vi "Corner Pixmap.vi"(10 "Corner":T2) -> (2 "Corner Pixmap":T1)   [LabVIEW 2022 SP3, in "FlexBlocks Support.lvlib"]
uses:
  FlexBlocks Support.lvlib
  <vilib>/picture/picture.llb/imagedata.ctl
  Corner.ctl
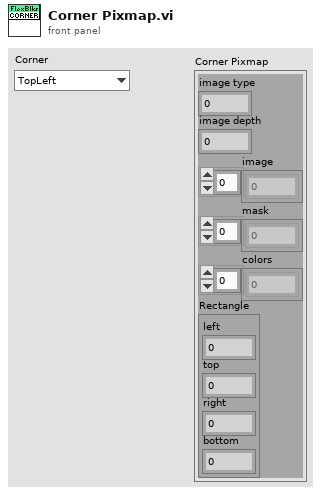
[diagram p1: front panel]
types:
  T1 = typedef "imagedata.ctl" = cluster{"image type":i32, "image depth":i32, "image":u8[], "mask":u8[], "colors":u32[], "Rectangle":cluster{"left":i16, "top":i16, "right":i16, "bottom":i16}}
  T2 = typedef "FlexBlocks Support.lvlib/Corner.ctl" = enum16{"TopLeft", "TopRight", "BottomLeft", "BottomRight"}
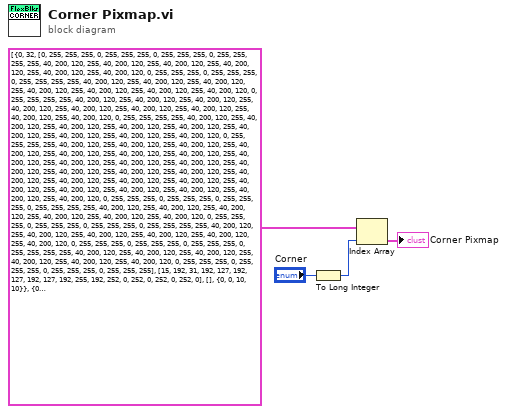
[diagram p0: block diagram]
diagram:
  n1 = To Long Integer(number="Corner") -> (32bit integer=w2:i32)
  n2 = Index Array(array=T1[] [{"image type"=0, "image depth"=32, "image"=[0, 255, 255, 255, 0, 255, 255, 255, 0, 255, 255, 255, 0, 255, 255, 255, 255, 40, 200, 120, 255, 40, 200, 120, 255, 40, 200, 120, 255, 40, 200, 120, 255, 40, 200, 120, 255, 40, 200, 120, 0, 255, 255, 255, 0, 255, 255, 255, 0, 255, 255, 255, 255, 40, 200, 120, 255, 40, 200, 120, 255, 40, 200, 120, 255, 40, 200, 120, 255, 40, 200, 120, 255, 40, 200, 120, 255, 40, 200, 120, 0, 255, 255, 255, 255, 40, 200, 120, 255, 40, 200, 120, 255, 40, 200, 120, 255, 40, 200, 120, 255, 40, 200, 120, 255, 40, 200, 120, 255, 40, 200, 120, 255, 40, 200, 120, 255, 40, 200, 120, 0, 255, 255, 255, 255, 40, 200, 120, 255, 40, 200, 120, 255, 40, 200, 120, 255, 40, 200, 120, 255, 40, 200, 120, 255, 40, 200, 120, 255, 40, 200, 120, 255, 40, 200, 120, 255, 40, 200, 120, 0, 255, 255, 255, 255, 40, 200, 120, 255, 40, 200, 120, 255, 40, 200, 120, 255, 40, 200, 120, 255, 40, 200, 120, 255, 40, 200, 120, 255, 40, 200, 120, 255, 40, 200, 120, 255, 40, 200, 120, 255, 40, 200, 120, 255, 40, 200, 120, 255, 40, 200, 120, 255, 40, 200, 120, 255, 40, 200, 120, 255, 40, 200, 120, 255, 40, 200, 120, 255, 40, 200, 120, 255, 40, 200, 120, 255, 40, 200, 120, 255, 40, 200, 120, 255, 40, 200, 120, 255, 40, 200, 120, 255, 40, 200, 120, 255, 40, 200, 120, 255, 40, 200, 120, 0, 255, 255, 255, 0, 255, 255, 255, 0, 255, 255, 255, 0, 255, 255, 255, 255, 40, 200, 120, 255, 40, 200, 120, 255, 40, 200, 120, 255, 40, 200, 120, 255, 40, 200, 120, 255, 40, 200, 120, 0, 255, 255, 255, 0, 255, 255, 255, 0, 255, 255, 255, 0, 255, 255, 255, 255, 40, 200, 120, 255, 40, 200, 120, 255, 40, 200, 120, 255, 40, 200, 120, 255, 40, 200, 120, 255, 40, 200, 120, 0, 255, 255, 255, 0, 255, 255, 255, 0, 255, 255, 255, 0, 255, 255, 255, 255, 40, 200, 120, 255, 40, 200, 120, 255, 40, 200, 120, 255, 40, 200, 120, 255, 40, 200, 120, 255, 40, 200, 120, 0, 255, 255, 255, 0, 255, 255, 255, 0, 255, 255, 255, 0, 255, 255, 255], "mask"=[15, 192, 31, 192, 127, 192, 127, 192, 127, 192, 255, 192, 252, 0, 252, 0, 252, 0, 252, 0], "colors"=[], "Rectangle"={"left"=0, "top"=0, "right"=10, "bottom"=10}}, {"image type"=0, "image depth"=32, "image"=[255, 40, 200, 120, 255, 40, 200, 120, 255, 40, 200, 120, 255, 40, 200, 120, 255, 40, 200, 120, 255, 40, 200, 120, 0, 255, 255, 255, 0, 255, 255, 255, 0, 255, 255, 255, 0, 255, 255, 255, 255, 40, 200, 120, 255, 40, 200, 120, 255, 40, 200, 120, 255, 40, 200, 120, 255, 40, 200, 120, 255, 40, 200, 120, 255, 40, 200, 120, 0, 255, 255, 255, 0, 255, 255, 255, 0, 255, 255, 255, 255, 40, 200, 120, 255, 40, 200, 120, 255, 40, 200, 120, 255, 40, 200, 120, 255, 40, 200, 120, 255, 40, 200, 120, 255, 40, 200, 120, 255, 40, 200, 120, 255, 40, 200, 120, 0, 255, 255, 255, 255, 40, 200, 120, 255, 40, 200, 120, 255, 40, 200, 120, 255, 40, 200, 120, 255, 40, 200, 120, 255, 40, 200, 120, 255, 40, 200, 120, 255, 40, 200, 120, 255, 40, 200, 120, 0, 255, 255, 255, 255, 40, 200, 120, 255, 40, 200, 120, 255, 40, 200, 120, 255, 40, 200, 120, 255, 40, 200, 120, 255, 40, 200, 120, 255, 40, 200, 120, 255, 40, 200, 120, 255, 40, 200, 120, 0, 255, 255, 255, 255, 40, 200, 120, 255, 40, 200, 120, 255, 40, 200, 120, 255, 40, 200, 120, 255, 40, 200, 120, 255, 40, 200, 120, 255, 40, 200, 120, 255, 40, 200, 120, 255, 40, 200, 120, 255, 40, 200, 120, 0, 255, 255, 255, 0, 255, 255, 255, 0, 255, 255, 255, 0, 255, 255, 255, 255, 40, 200, 120, 255, 40, 200, 120, 255, 40, 200, 120, 255, 40, 200, 120, 255, 40, 200, 120, 255, 40, 200, 120, 0, 255, 255, 255, 0, 255, 255, 255, 0, 255, 255, 255, 0, 255, 255, 255, 255, 40, 200, 120, 255, 40, 200, 120, 255, 40, 200, 120, 255, 40, 200, 120, 255, 40, 200, 120, 255, 40, 200, 120, 0, 255, 255, 255, 0, 255, 255, 255, 0, 255, 255, 255, 0, 255, 255, 255, 255, 40, 200, 120, 255, 40, 200, 120, 255, 40, 200, 120, 255, 40, 200, 120, 255, 40, 200, 120, 255, 40, 200, 120, 0, 255, 255, 255, 0, 255, 255, 255, 0, 255, 255, 255, 0, 255, 255, 255, 255, 40, 200, 120, 255, 40, 200, 120, 255, 40, 200, 120, 255, 40, 200, 120, 255, 40, 200, 120, 255, 40, 200, 120], "mask"=[252, 0, 254, 0, 255, 128, 255, 128, 255, 128, 255, 192, 15, 192, 15, 192, 15, 192, 15, 192], "colors"=[], "Rectangle"={"left"=0, "top"=0, "right"=10, "bottom"=10}}, {"image type"=0, "image depth"=32, "image"=[255, 40, 200, 120, 255, 40, 200, 120, 255, 40, 200, 120, 255, 40, 200, 120, 255, 40, 200, 120, 255, 40, 200, 120, 0, 255, 255, 255, 0, 255, 255, 255, 0, 255, 255, 255, 0, 255, 255, 255, 255, 40, 200, 120, 255, 40, 200, 120, 255, 40, 200, 120, 255, 40, 200, 120, 255, 40, 200, 120, 255, 40, 200, 120, 0, 255, 255, 255, 0, 255, 255, 255, 0, 255, 255, 255, 0, 255, 255, 255, 255, 40, 200, 120, 255, 40, 200, 120, 255, 40, 200, 120, 255, 40, 200, 120, 255, 40, 200, 120, 255, 40, 200, 120, 0, 255, 255, 255, 0, 255, 255, 255, 0, 255, 255, 255, 0, 255, 255, 255, 255, 40, 200, 120, 255, 40, 200, 120, 255, 40, 200, 120, 255, 40, 200, 120, 255, 40, 200, 120, 255, 40, 200, 120, 0, 255, 255, 255, 0, 255, 255, 255, 0, 255, 255, 255, 0, 255, 255, 255, 255, 40, 200, 120, 255, 40, 200, 120, 255, 40, 200, 120, 255, 40, 200, 120, 255, 40, 200, 120, 255, 40, 200, 120, 255, 40, 200, 120, 255, 40, 200, 120, 255, 40, 200, 120, 255, 40, 200, 120, 255, 40, 200, 120, 255, 40, 200, 120, 255, 40, 200, 120, 255, 40, 200, 120, 255, 40, 200, 120, 255, 40, 200, 120, 255, 40, 200, 120, 255, 40, 200, 120, 255, 40, 200, 120, 255, 40, 200, 120, 0, 255, 255, 255, 255, 40, 200, 120, 255, 40, 200, 120, 255, 40, 200, 120, 255, 40, 200, 120, 255, 40, 200, 120, 255, 40, 200, 120, 255, 40, 200, 120, 255, 40, 200, 120, 255, 40, 200, 120, 0, 255, 255, 255, 0, 255, 255, 255, 255, 40, 200, 120, 255, 40, 200, 120, 255, 40, 200, 120, 255, 40, 200, 120, 255, 40, 200, 120, 255, 40, 200, 120, 255, 40, 200, 120, 255, 40, 200, 120, 0, 255, 255, 255, 0, 255, 255, 255, 255, 40, 200, 120, 255, 40, 200, 120, 255, 40, 200, 120, 255, 40, 200, 120, 255, 40, 200, 120, 255, 40, 200, 120, 255, 40, 200, 120, 255, 40, 200, 120, 0, 255, 255, 255, 0, 255, 255, 255, 0, 255, 255, 255, 0, 255, 255, 255, 0, 255, 255, 255, 255, 40, 200, 120, 255, 40, 200, 120, 255, 40, 200, 120, 255, 40, 200, 120, 255, 40, 200, 120], "mask"=[252, 0, 252, 0, 252, 0, 252, 0, 255, 192, 255, 192, 127, 192, 63, 192, 63, 192, 7, 192], "colors"=[], "Rectangle"={"left"=0, "top"=0, "right"=10, "bottom"=10}}, {"image type"=0, "image depth"=32, "image"=[0, 255, 255, 255, 0, 255, 255, 255, 0, 255, 255, 255, 0, 255, 255, 255, 0, 255, 255, 255, 0, 255, 255, 255, 0, 255, 255, 255, 0, 255, 255, 255, 0, 255, 255, 255, 0, 255, 255, 255, 0, 255, 255, 255, 0, 255, 255, 255, 0, 255, 255, 255, 0, 255, 255, 255, 0, 255, 255, 255, 0, 255, 255, 255, 0, 255, 255, 255, 0, 255, 255, 255, 0, 255, 255, 255, 0, 255, 255, 255, 0, 255, 255, 255, 0, 255, 255, 255, 255, 40, 200, 120, 255, 40, 200, 120, 255, 40, 200, 120, 255, 40, 200, 120, 255, 40, 200, 120, 255, 40, 200, 120, 255, 40, 200, 120, 255, 40, 200, 120, 0, 255, 255, 255, 0, 255, 255, 255, 0, 255, 255, 255, 255, 40, 200, 120, 255, 40, 200, 120, 255, 40, 200, 120, 255, 40, 200, 120, 255, 40, 200, 120, 255, 40, 200, 120, 255, 40, 200, 120, 255, 40, 200, 120, 255, 40, 200, 120, 255, 40, 200, 120, 255, 40, 200, 120, 255, 40, 200, 120, 255, 40, 200, 120, 255, 40, 200, 120, 255, 40, 200, 120, 255, 40, 200, 120, 255, 40, 200, 120, 255, 40, 200, 120, 255, 40, 200, 120, 255, 40, 200, 120, 255, 40, 200, 120, 255, 40, 200, 120, 255, 40, 200, 120, 255, 40, 200, 120, 255, 40, 200, 120, 255, 40, 200, 120, 255, 40, 200, 120, 255, 40, 200, 120, 255, 40, 200, 120, 255, 40, 200, 120, 255, 40, 200, 120, 255, 40, 200, 120, 255, 40, 200, 120, 255, 40, 200, 120, 255, 40, 200, 120, 255, 40, 200, 120, 255, 40, 200, 120, 255, 40, 200, 120, 255, 40, 200, 120, 255, 40, 200, 120, 255, 40, 200, 120, 255, 40, 200, 120, 255, 40, 200, 120, 255, 40, 200, 120, 255, 40, 200, 120, 255, 40, 200, 120, 255, 40, 200, 120, 255, 40, 200, 120, 255, 40, 200, 120, 255, 40, 200, 120, 255, 40, 200, 120, 255, 40, 200, 120, 255, 40, 200, 120, 255, 40, 200, 120, 255, 40, 200, 120, 255, 40, 200, 120, 255, 40, 200, 120, 255, 40, 200, 120, 255, 40, 200, 120, 255, 40, 200, 120, 255, 40, 200, 120, 255, 40, 200, 120, 255, 40, 200, 120, 0, 255, 255, 255, 0, 255, 255, 255, 0, 255, 255, 255, 255, 40, 200, 120], "mask"=[0, 0, 0, 0, 63, 192, 31, 192, 255, 192, 255, 192, 255, 192, 255, 192, 255, 192, 252, 64], "colors"=[], "Rectangle"={"left"=0, "top"=0, "right"=10, "bottom"=10}}], index=w2) -> (element=→"Corner Pixmap":T1)
